vi "Read Output.vi"(8 "error in (no error)":errorcluster, 11 "CallEXEStep in":refnum<class "CallEXEStep.lvclass">) -> (0 "error out":errorcluster, 2 "Output":T1[](array[typedef]), 3 "CallEXEStep out":refnum<class "CallEXEStep.lvclass">)   [LabVIEW 2015, in "CallEXEStep.lvclass"]
uses:
  CallEXEStep.lvclass
  Step/STEP_OUTPUT.ctl
  Step/OUTPUT_DATA_TYPE.ctl
  OutputUI/OUTPUT_CHECK_TYPE.ctl
  Step/OUTPUT_VALUE_TYPE.ctl
  Step.lvclass
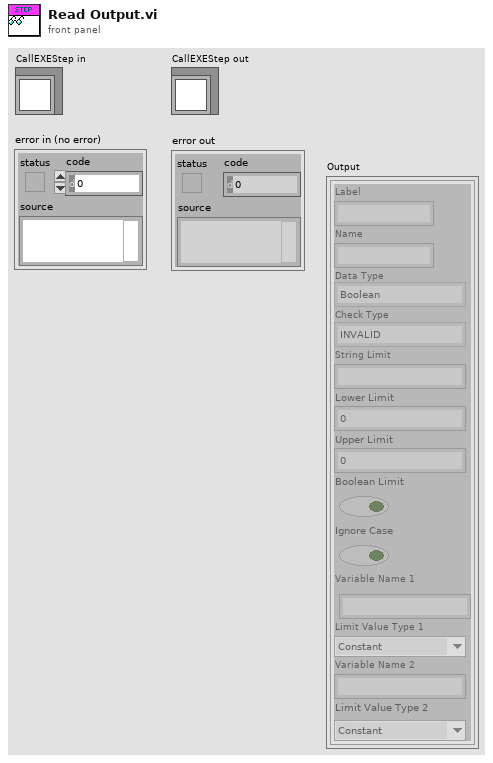
[diagram p1: front panel]
types:
  T1 = typedef "Step.lvclass/STEP_OUTPUT.ctl" = cluster{"Label":string, "Name":string, "Data Type":T2, "Check Type":T3, "String Limit":string, "Lower Limit":dbl, "Upper Limit":dbl, "Boolean Limit":bool, "Ignore Case":bool, "Variable Name 1":string, "Limit Value Type 1":T4, "Variable Name 2":string, "Limit Value Type 2":T4}
  T2 = typedef "Step.lvclass/OUTPUT_DATA_TYPE.ctl" = enum16{"Boolean", "String", "Numeric", "Other"}
  T3 = typedef "Step.lvclass/OUTPUT_CHECK_TYPE.ctl" = enum16{"INVALID", "DO_NOT_CHECK", "RECORD", "VARIABLE", "EQUAL", "NOT_EQUAL", "STR_CONTAINS", "STR_START_WITH", "STR_END_WITH", "STR_REGEX_MATCH", "NUM_GT", "NUM_LT", "NUM_GE", "NUM_LE", "NUM_RANGE", "NUM_RANGE_BDY"}
  T4 = typedef "Step.lvclass/OUTPUT_VALUE_TYPE.ctl" = enum16{"Constant", "Variable"}
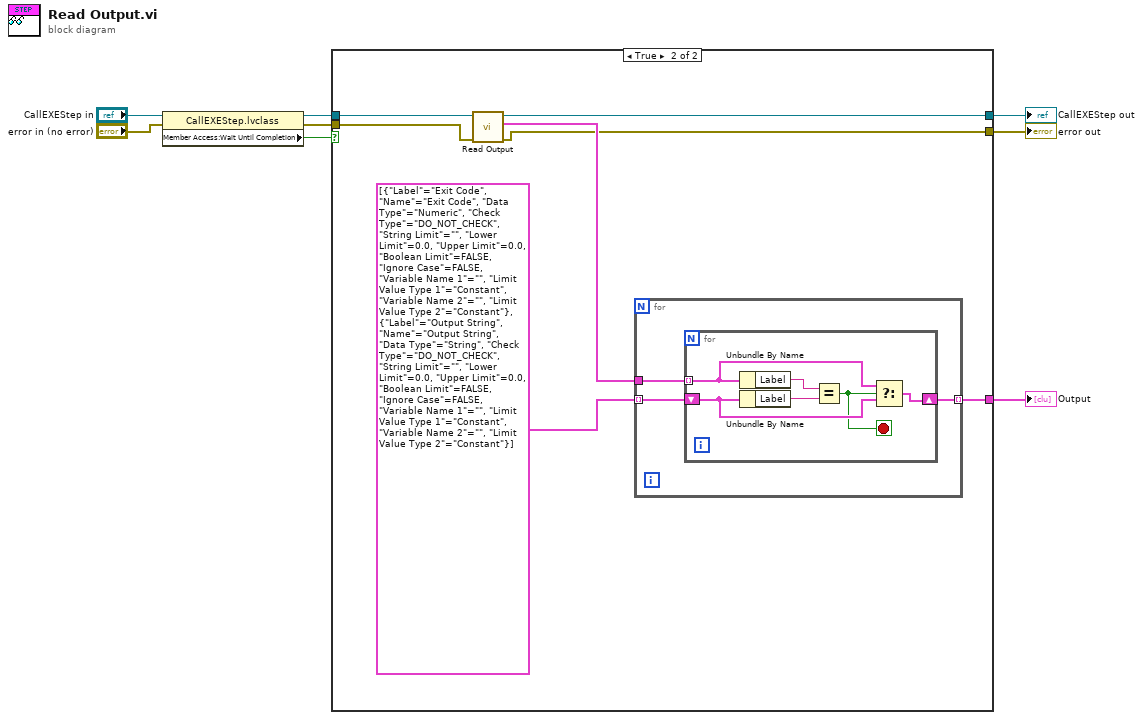
[diagram p0: block diagram]
diagram:
  n1 = property class="CallEXEStep.lvclass"(reference="CallEXEStep in", error in="error in (no error)") -> (reference out=w4:refnum<class "CallEXEStep.lvclass">, error out=w2:errorcluster, "Member Access:Wait Until Completion"=w1:bool)
  n2 = case shown="True" w1 {
    tunnel: [_ w15] -> w8
    tunnel: [w9 w14] -> w7
    tunnel: [w10 w13] -> w6
    tunnel: w4 -> [w10 w12]
    tunnel: w2 -> [w9 w11]
    frame False {
    }
    frame True {
      n3 = call-parent "Read Output.vi"("error in (no error)"=w11, "Step in"=w12) -> ("error out"=w14:errorcluster, "Output"=w17:T1[], "Step out"=w13:refnum<class "CallEXEStep.lvclass">)  [unwired: 7 in]
      n4 = for {
        tunnel: T1[] [{"Label"="Exit Code", "Name"="Exit Code", "Data Type"=enum."Numeric", "Check Type"=enum."DO_NOT_CHECK", "String Limit"="", "Lower Limit"=0.0, "Upper Limit"=0.0, "Boolean Limit"=FALSE, "Ignore Case"=FALSE, "Variable Name 1"="", "Limit Value Type 1"=enum."Constant", "Variable Name 2"="", "Limit Value Type 2"=enum."Constant"}, {"Label"="Output String", "Name"="Output String", "Data Type"=enum."String", "Check Type"=enum."DO_NOT_CHECK", "String Limit"="", "Lower Limit"=0.0, "Upper Limit"=0.0, "Boolean Limit"=FALSE, "Ignore Case"=FALSE, "Variable Name 1"="", "Limit Value Type 1"=enum."Constant", "Variable Name 2"="", "Limit Value Type 2"=enum."Constant"}] ("Output") -> [w19] mode=indexing
        tunnel: w17 -> [w20]
        tunnel: [w18] -> w15 mode=indexing
        n5 = for {
          tunnel: w20 -> [w24] mode=indexing
          shift-right: [w22] -> w18
          shift-left: w19 -> [w23]
          stop <- w21 stop-if-true
          n6 = Unbundle By Name(w24) -> ("Label"=w25:string)
          n7 = Unbundle By Name(w23) -> ("Label"=w26:string)
          n8 = Equal?(x=w25, y=w26) -> (x = y?=w21:bool)
          n9 = Select(t=w24, s=w21, f=w23) -> (s? t:f=w22:T1)
        }
      }
    }
  }
  "error out" <- w7
  "CallEXEStep out" <- w6
  "Output" <- w8
